vi "Module Error.vi"(8 "error in":errorcluster, 11 "Module Error In":errorcluster) -> (0 "error out":errorcluster, 3 "Module Error Out":errorcluster)   [LabVIEW 2015, in "Generic Module Library.lvlib" / "Template G_Module.lvlib"]
uses:
  Template G_Module.lvlib
  Private Controls/Event Item.ctl
  Broadcast Support/Broadcast Actions.ctl
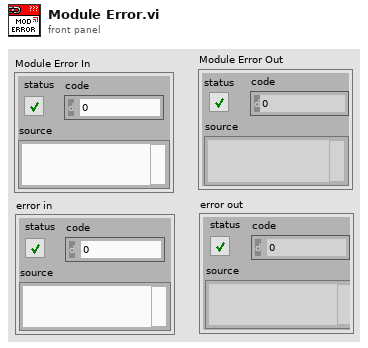
[diagram p1: front panel]
types:
  T1 = typedef "Generic Module Library.lvlib/Template G_Module.lvlib/Broadcast Actions.ctl" = enum16{"Create", "Get", "Destroy"}
  T2 = typedef "Generic Module Library.lvlib/Template G_Module.lvlib/Event Item.ctl" = cluster{"Event Data":variant}
  T3 = typedef "Generic Module Library.lvlib/Template G_Module.lvlib/Broadcast List.ctl" = cluster{"Module Started":refnum<user-event>, "Module Error":refnum<user-event>, "Module Pong":refnum<user-event>, "Module Status":refnum<user-event>, "Module Stopping":refnum<user-event>, "Module Stopped":refnum<user-event>, "Module Reinitialized":refnum<user-event>}
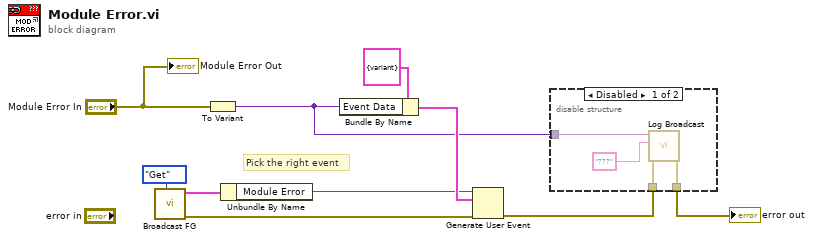
[diagram p0: block diagram]
diagram:
  # "Pick the right event"
  n1 = call "Broadcast FG.vi"("Broadcast Actions"=Broadcast_Actions."Get") -> ("error out"=w10:errorcluster, "Broadcast List"=w5:T3)  [unwired: 9 in]
  n2 = To Variant(anything="Module Error In") -> (Variant=w1:variant)
  n3 = Unbundle By Name(w5) -> ("Module Error"=w6:refnum<user-event>)
  n4 = Bundle By Name(cluster=T2 {"Event Data"=variant} ("Broadcast Item"), "Event Data"=w1) -> (w8:T2)
  n5 = Generate User Event(user event=w6, event data cluster=w8, error in=w10) -> (error out=w3:errorcluster)  [unwired: 1 in, 1 out]
  n6 = disable-structure shown="Disabled" {
    disable-tunnel: w3 -> [w14 w15]
    disable-tunnel: [w13 w15] -> w2
    disable-tunnel: w1 -> [w11 _]
    frame Disabled {
      n7 = call "Log Broadcast.vi"("error in"=w14, "Broadcast Name"="???", "Message Data In"=w11) -> ("error out"=w13:errorcluster)  [unwired: 8 in]
    }
    frame Enabled {
    }
  }
  "error out" <- w2
  "Module Error Out" <- "Module Error In"
